vi "Climb_Pivot_Execute.vi"() -> ()   [LabVIEW 2019]
uses:
  Climb_Globals.vi
  <vilib>/Rock Robotics/WPI/ThirdParty/REV Robotics/SPARK MAX/Typedef/Spark MAX Control Type.ctl
  Globals/Sensor_Values.vi
  Climb_Pivot_Control_States.ctl
  Climb_Pivot_Cluster.ctl
panel:
  in  "Climb_Pivot_Limit":dbl=-64.0
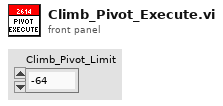
[diagram p1: front panel]
types:
  T1 = typedef "WPI_MotorControlDeviceRef.ctl" = cluster{"DeviceStatus":errorcluster, "Type":T2, "PWM":cluster{"PWM Channel":T3, "DeadBand":T4}, "CAN":cluster{"Device Number":u8, "SetOutput VI Ref":variant, "GetOutput VI Ref":variant, "Enable VI Ref":variant, "Disable VI Ref":variant, "Data":variant}, "Invert":bool, "DIO PWM":cluster{"PWM \"Enable\" Channel":T3, "DIOChannel":T5, "PWM Rate":dbl}}
  T2 = typedef "WPI_MotorControlType.ctl" = enum16{"PWM", "CAN", "DIO PWM"}
  T3 = typedef "FPGA_DIOPWMChannel.ctl" = enum8{"PWM 0", "PWM 1", "PWM 2", "PWM 3", "PWM 4", "PWM 5", "PWM 6", "PWM 7", "PWM 8", "PWM 9", "PWM MXP 0", "PWM MXP 1", "PWM MXP 2", "PWM MXP 3", "PWM MXP 4", "PWM MXP 5", "PWM MXP 6", "PWM MXP 7", "PWM MXP 8", "PWM MXP 9", "Invalid"}
  T4 = typedef "WPI_PWMDeadband.ctl" = cluster{"Name":string, "maxPositivePwm":i32, "minPositivePwm":i32, "centerPwm":i32, "maxNegativePwm":i32, "minNegativePwm":i32, "angularRange":u16}
  T5 = typedef "FPGA_DIOChannel.ctl" = enum8{"DIO 0", "DIO 1", "DIO 2", "DIO 3", "DIO 4", "DIO 5", "DIO 6", "DIO 7", "DIO 8", "DIO 9", "DIO MXP 0", "DIO MXP 1", "DIO MXP 2", "DIO MXP 3", "DIO MXP 4", "DIO MXP 5", "DIO MXP 6", "DIO MXP 7", "DIO MXP 8", "DIO MXP 9", "DIO MXP 10", "DIO MXP 11", "DIO MXP 12", "DIO MXP 13", "DIO MXP 14", "DIO MXP 15", "SPI Port CS1", "SPI Port CS2", "SPI Port CS3", "SPI Port MISO", "SPI Port MOSI", "Invalid"}
  T6 = typedef "Climb_Pivot_Cluster.ctl" = cluster{"Up?":bool, "Pivot_Throttle":dbl, "Control_States":T7}
  T7 = typedef "Climb_Pivot_Control_States.ctl" = enum16{"No-Op", "Moving_Down", "Moving_Up", "Manual"}
  T8 = typedef "Spark MAX Control Type.ctl" = enum16{"Percent VBus", "Voltage", "Velocity", "Position", "Smart Motion", "Current", "Smart Velocity"}
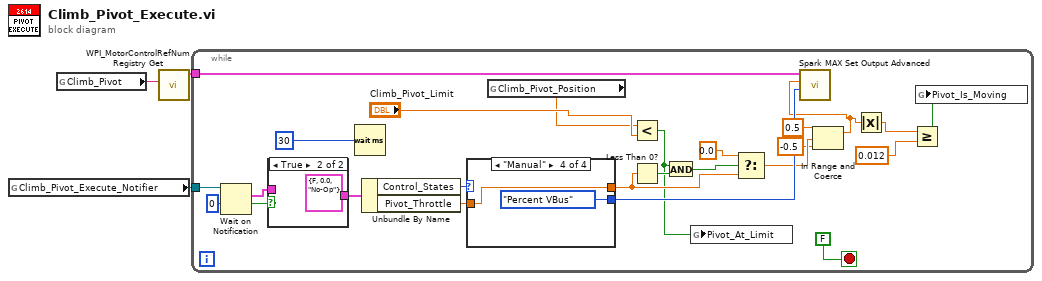
[diagram p0: block diagram]
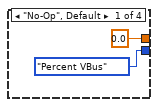
[diagram p3: hidden frame]
diagram:
  n1 = global read "Climb_Globals.vi" "Climb_Pivot_Execute_Notifier"() -> (w3:refnum<notifier>)
  n2 = global read "Climb_Globals.vi" "Climb_Pivot"() -> (w2:string)
  n3 = call <vilib>:"WPI_MotorControlRefNum Registry Get.vi"("refnum name"=w2) -> ("MotorControlDevRef"=w1:T1)  [unwired: 9 in, 1 out]
  n4 = while {
    tunnel: w3 -> [w27]
    tunnel: w1 -> [w25]
    stop <- FALSE stop-if-true
    n5 = Wait on Notification(notifier=w27, timeout in ms (-1)=0) -> (notification=w12:T6, timed out?=w13:bool)  [unwired: 2 in, 2 out]
    n6 = case shown="True" w13 {
      tunnel: w12 -> [w29 _]
      tunnel: [w29 T6 {"Up?"=FALSE, "Pivot_Throttle"=0.0, "Control_States"=enum."No-Op"} ("Climb_Pivot_Cluster")] -> w11
      frame False {
      }
      frame True {
      }
    }
    n7 = Wait (ms)(milliseconds to wait=u32 30) -> ()  [unwired: 1 out]
    n8 = Unbundle By Name(w11) -> ("Control_States"=w26:T7, "Pivot_Throttle"=w23:dbl)
    n9 = case shown="\"Manual\"" w26 {
      tunnel: [0.0 ("Arbitrary Feed Forward (0)") _ _ w33] -> w21
      tunnel: [Spark_MAX_Control_Type."Percent VBus" ("Control Mode") _ _ Spark_MAX_Control_Type."Percent VBus" ("Control Mode")] -> w24
      tunnel: w23 -> [_ _ _ w33]
      frame "No-Op", Default {
      }
      frame "Moving_Down" {
      }
      frame "Moving_Up" {
      }
      frame "Manual" {
      }
    }
    n10 = global read "Sensor_Values.vi" "Climb_Pivot_Position"() -> (w9:dbl)
    n11 = Less?(x=w9, y="Climb_Pivot_Limit") -> (x < y?=w8:bool)
    n12 = Less Than 0?(x=w21) -> (x < 0?=w22:bool)
    n13 = And(x=w8, y=w22) -> (x .and. y?=w20:bool)
    n14 = global write "Climb_Globals.vi" "Pivot_At_Limit"(w8) -> ()
    n15 = Select(t=0.0, s=w20, f=w21) -> (s? t:f=w18:dbl)
    n16 = In Range and Coerce(upper limit=0.5, x=w18, lower limit=-0.5) -> (coerced(x)=w7:dbl)  [unwired: 1 out]
    n17 = call <vilib>:"Spark MAX Set Output Advanced.vi"("Control Mode"=w24, "Setpoint"=w7, "MotorControlDevRef"=w25) -> ()  [unwired: 7 in, 2 out]
    n18 = Absolute Value(x=w7) -> (abs(x)=w5:dbl)
    n19 = Greater Or Equal?(x=w5, y=0.012) -> (x >= y?=w4:bool)
    n20 = global write "Climb_Globals.vi" "Pivot_Is_Moving"(w4) -> ()
  }
